vi "closeHandler.vi"(8 "error in (no error)":errorcluster, 11 "Handler.UserEvent.Console in":refnum<class "Handler.UserEvent.Console.lvclass">) -> (0 "error out":errorcluster, 3 "Handler.UserEvent.Console out":refnum<class "Handler.UserEvent.Console.lvclass">)   [LabVIEW 2017, in "Error Log.lvlib" / "Handler.UserEvent.Console.lvclass"]
uses:
  Handler.UserEvent.Console.lvclass
  Handler.UserEvent/Handler.UserEvent.lvclass
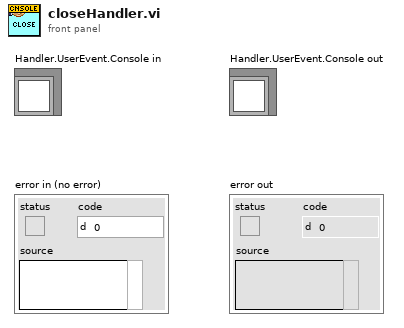
[diagram p1: front panel]
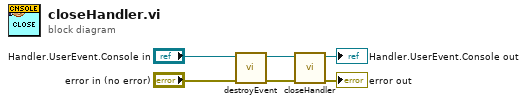
[diagram p0: block diagram]
diagram:
  n1 = call-dynamic "destroyEvent.vi"("error in (no error)"="error in (no error)", "Handler.UserEvent.Console in"="Handler.UserEvent.Console in") -> ("error out"=w1:errorcluster, "Handler.UserEvent.Console out"=w2:refnum<class "Handler.UserEvent.Console.lvclass">)  [unwired: 8 in]
  n2 = call-parent "closeHandler.vi"("error in (no error)"=w1, "Handler.UserEvent in"=w2) -> ("error out"=→"error out":errorcluster, "Handler.UserEvent out"=→"Handler.UserEvent.Console out":refnum<class "Handler.UserEvent.Console.lvclass">)  [unwired: 8 in]
